vi "Step Add.vi"(8 "error in (no error)":errorcluster, 10 "Step Record":T1, 11 "Connection Refnum":T2) -> (0 "error out":errorcluster, 2 "New Step Record":T1, 3 "Connection Refnum":T2)   [LabVIEW 2011]
uses:
  Step Record.ctl
  SI.LIB/ODBC/SQL Controls/Connection Refnum.ctl
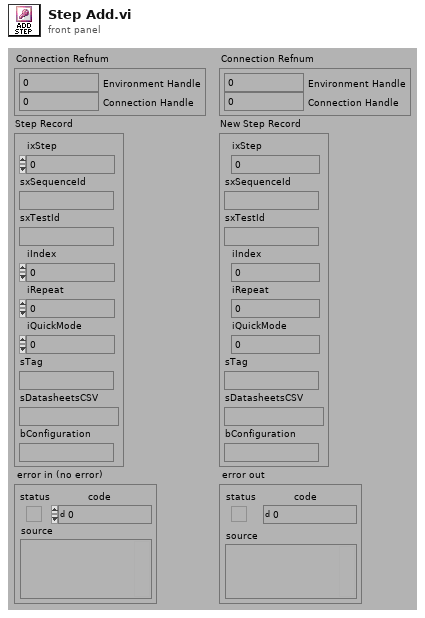
[diagram p1: front panel]
types:
  T1 = typedef "Step Record.ctl" = cluster{"ixStep":i32, "sxSequenceId":string, "sxTestId":string, "iIndex":i32, "iRepeat":i32, "iQuickMode":i32, "sTag":string, "sDatasheetsCSV":string, "bConfiguration":string}
  T2 = typedef "Connection Refnum.ctl" = cluster{"Environment Handle":i32, "Connection Handle":i32}
  T3 = typedef "Statement Refnum.ctl" = cluster{"Statement Handle":i32, "Parameter Number":u16}
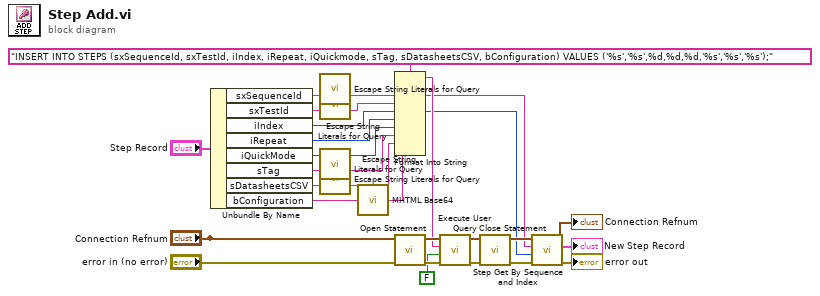
[diagram p0: block diagram]
diagram:
  n1 = Unbundle By Name("Step Record") -> ("sxSequenceId"=w19:string, "sxTestId"=w18:string, "iIndex"=w1:i32, "iRepeat"=w16:i32, "iQuickMode"=w15:i32, "sTag"=w14:string, "sDatasheetsCSV"=w12:string, "bConfiguration"=w10:string)
  n2 = call "Escape String Literals for Query.vi"("String"=w19) -> ("escaped String"=w2:string)  [unwired: 1 in, 13 out]
  n3 = call "Escape String Literals for Query.vi"("String"=w18) -> ("escaped String"=w17:string)  [unwired: 1 in, 13 out]
  n4 = call "Escape String Literals for Query.vi"("String"=w14) -> ("escaped String"=w13:string)  [unwired: 1 in, 13 out]
  n5 = call "Escape String Literals for Query.vi"("String"=w12) -> ("escaped String"=w11:string)  [unwired: 1 in, 13 out]
  n6 = call "MHTML Base64.vi"("Binary String"=w10) -> ("String (Base64)"=w9:string)  [unwired: 14 out]
  n7 = Format Into String(format string="INSERT INTO STEPS (sxSequenceId, sxTestId, iIndex, iRepeat, iQuickmode, sTag, sDatasheetsCSV, bConfiguration) VALUES ('%s','%s',%d,%d,%d,'%s','%s','%s');" ("User Query"), w2, w17, w1, w16, w15, w13, w11, w9) -> (resulting string=w21:string)  [unwired: 2 in, 1 out]
  n8 = call "Open Statement.vi"("error in (no error)"="error in (no error)", "Connection Refnum"="Connection Refnum") -> ("error out"=w23:errorcluster, "Statement Refnum"=w22:T3)  [unwired: 4 out]
  n9 = call "Execute User Query.vi"("error in (no error)"=w23, "Return Data? (f)"=FALSE, "User Query"=w21, "Statement Refnum"=w22) -> ("error out"=w24:errorcluster, "Statement Refnum"=w25:T3)  [unwired: 2 out]
  n10 = call "Close Statement.vi"("error in (no error)"=w24, "Statement Refnum"=w25) -> ("error out"=w7:errorcluster)  [unwired: 5 out]
  n11 = call "Step Get By Sequence and Index.vi"("error in (no error)"=w7, "iIndex"=w1, "sxSequenceID"=w2, "Connection Refnum"="Connection Refnum") -> ("error out"=→"error out":errorcluster, "Step Record"=→"New Step Record":T1, "Connection Refnum"=→"Connection Refnum":T2)  [unwired: 4 in, 1 out]
